vi "注册.vi"(8 "error in (no error)":errorcluster caption="错误输入（无错误）", 11 "Key Number":string="10") -> (0 "error out":errorcluster caption="错误输出")   [LabVIEW 2017]
uses:
  <vilib>/registry/registry.llb/Registry RtKey.ctl
  <vilib>/registry/registry.llb/Write Registry Value Simple.vi
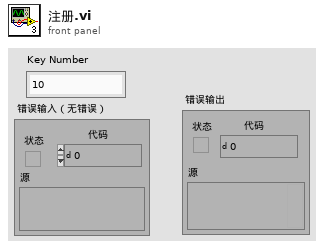
[diagram p1: front panel]
types:
  T1 = typedef "Registry RtKey.ctl" = enum32{"HKEY_CLASSES_ROOT", "HKEY_CURRENT_USER", "HKEY_LOCAL_MACHINE", "HKEY_USERS", "HKEY_PERFORMANCE_DATA", "HKEY_CURRENT_CONFIG", "HKEY_DYN_DATA"}
  T2 = typedef "Registry refnum.ctl" = refnum<k1>
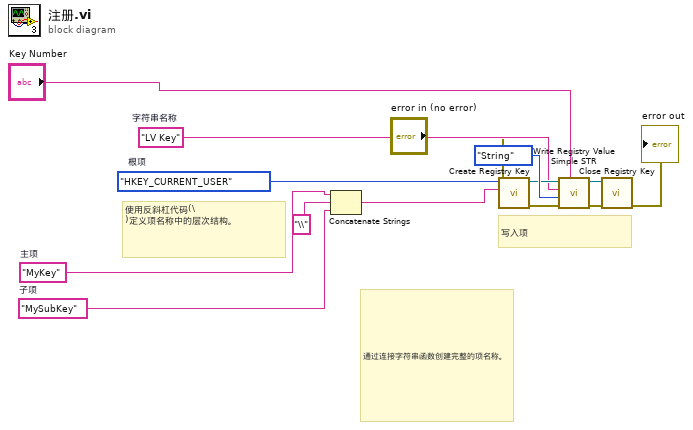
[diagram p0: block diagram]
diagram:
  w3 = "MySubKey"  # 子项
  w4 = "MyKey"  # 主项
  w7 = "LV Key"  # 字符串名称
  w9 = Registry_RtKey."HKEY_CURRENT_USER"  # 根项
  # "通过连接字符串函数创建完整的项名称。"
  # "使用反斜杠代码(\\)定义项名称中的层次结构。"
  # "写入项"
  n1 = Concatenate Strings(w4, "\\", w3) -> (w8:string)
  n2 = call <vilib>:"Create Registry Key.vi"("error in (no error)"="error in (no error)", "subkey"=w8, "root key (HKEY_LOCAL_MACHINE)"=w9) -> ("error out"=w12:errorcluster, "refnum out"=w10:T2)  [unwired: 6 in, 1 out]
  n3 = call-poly <vilib>:"Write Registry Value Simple STR.vi"("String/Binary data"="Key Number", "error in (no error)"=w12, "simple data type"=enum16{"String", "Binary", "DWORD"}."String", "value"=w7, "refnum"=w10) -> ("error out"=w14:errorcluster, "refnum out"=w13:T2)  [unwired: 3 in]
  n4 = call <vilib>:"Close Registry Key.vi"("error in (no error)"=w14, "refnum"=w13) -> ("error out"=→"error out":errorcluster)  [unwired: 5 in]
